vi "Ramp Slow.vi"(8 "error in (no error)":errorcluster, 9 "fieldIN":dbl[unit] caption="Field", 10 "Rate":dbl[unit], 11 "Power Supply in":refnum<class "Power Supply.lvclass">) -> (0 "error out":errorcluster, 1 "Rate Out":dbl[unit], 3 "Power Supply out":refnum<class "Power Supply.lvclass">)   [LabVIEW 2009, in "Power Supply.lvclass"]
uses:
  Power Supply.lvclass
  Power Supply.lvclass/Power Supply.ctl
panel:
  out "Training Cluster":T1
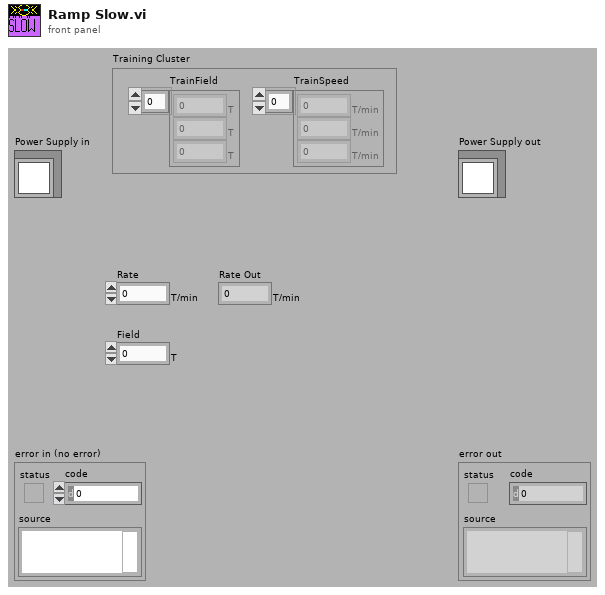
[diagram p1: front panel]
types:
  T1 = cluster{"TrainField":dbl[unit][], "TrainSpeed":dbl[unit][]}
  T2 = cluster{"Training Field":dbl[unit][], "Training Speed":dbl[unit][]}
  T3 = typedef "PSIO.ctl" = cluster{"Address":T4, "Version":enum16{"PS", "IPS"}}
  T4 = typedef "OxfordAddress.ctl" = cluster{"Com Port":i32, "ISOBUS Address":i32, "GPIB Address":i16, "Communication":enum16{"RS232", "ISOBUS", "GPIB", "Gateway"}}
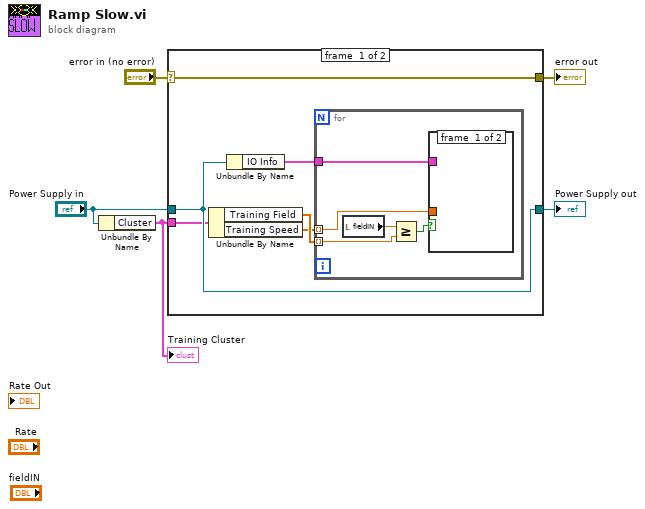
[diagram p0: block diagram]
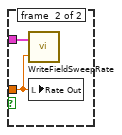
[diagram p2: hidden frame]
diagram:
  n1 = Unbundle By Name("Power Supply in") -> ("Cluster"=w1:T2)
  "Training Cluster" <- w1
  n2 = case shown="No Error" "error in (no error)" {
    selector: "error in (no error)" -> [w7 w19]
    tunnel: [w7 w19] -> w4
    tunnel: "Power Supply in" -> [w11 w20]
    tunnel: [w11 w20] -> w3
    tunnel: w1 -> [w6 _]
    frame #0 {
      n3 = Unbundle By Name(w6) -> ("Training Field"=w10:dbl[unit][], "Training Speed"=w8:dbl[unit][])
      n4 = Unbundle By Name(w11) -> ("IO Info"=w9:T3)
      n5 = for {
        tunnel: w10 -> [w15] mode=indexing
        tunnel: w9 -> [w13]
        tunnel: w8 -> [w12] mode=indexing
        n6 = local read "fieldIN"() -> (w16:dbl[unit])
        n7 = Greater Or Equal?(x=w16, y=w15) -> (x >= y?=w14:bool)
        n8 = case shown="True" w14 {
          tunnel: w13 -> [_ w18]
          tunnel: w12 -> [_ w17]
          frame #0 {
          }
          frame #1 {
            n9 = call "WriteFieldSweepRate.vi"("Sweep rate"=w17, "IO Info"=w18) -> ()  [unwired: 1 out]
            n10 = local write "Rate Out"(w17) -> ()
          }
        }
      }
    }
    frame #1 {
    }
  }
  "error out" <- w4
  "Power Supply out" <- w3
